vi "Set SubPnl Ref.vi"(10 "SubPnl Ref":refnum<vi>, 11 "Study Actor in":refnum<class "Study Actor.lvclass">) -> (3 "Study Actor out":refnum<class "Study Actor.lvclass">)   [LabVIEW 2024, in "Study Actor.lvlib" / "Study Actor.lvclass"]
uses:
  Study Actor.lvclass
  Study Actor.lvclass/Study Actor.ctl
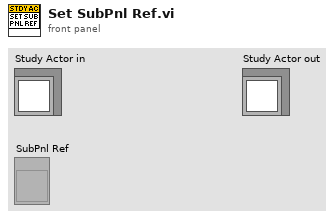
[diagram p1: front panel]
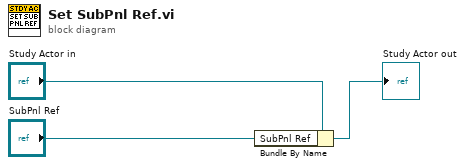
[diagram p0: block diagram]
diagram:
  n1 = Bundle By Name(cluster="Study Actor in", "SubPnl Ref"="SubPnl Ref") -> (→"Study Actor out":refnum<class "Study Actor.lvclass">)
